vi "Read TDMS waveform --V3.vi"(0 "Input file path":path, 1 "tdms file in":refnum<k34>, 2 "TDMS":T1, 5 "Data window IN":T2={"Start"=39994, "Length"=13169, "Channel numbers"=[0], "Cannel names"=["freq", ""], "Group name"="p"}, 11 "error in":errorcluster) -> (3 "tdms file out":refnum<k34>, 4 "Actual input file path":path, 6 "Data out":waveform(dbl)[](array[waveform]), 8 "All Data out":waveform(dbl)[](array[waveform]), 10 "1st channel length":u64, 15 "error out":errorcluster)   [LabVIEW 2021]
uses:
  fft -- data win.ctl
  Read TDMS waveform -- control.vi.ctl
panel:
  # "OR"
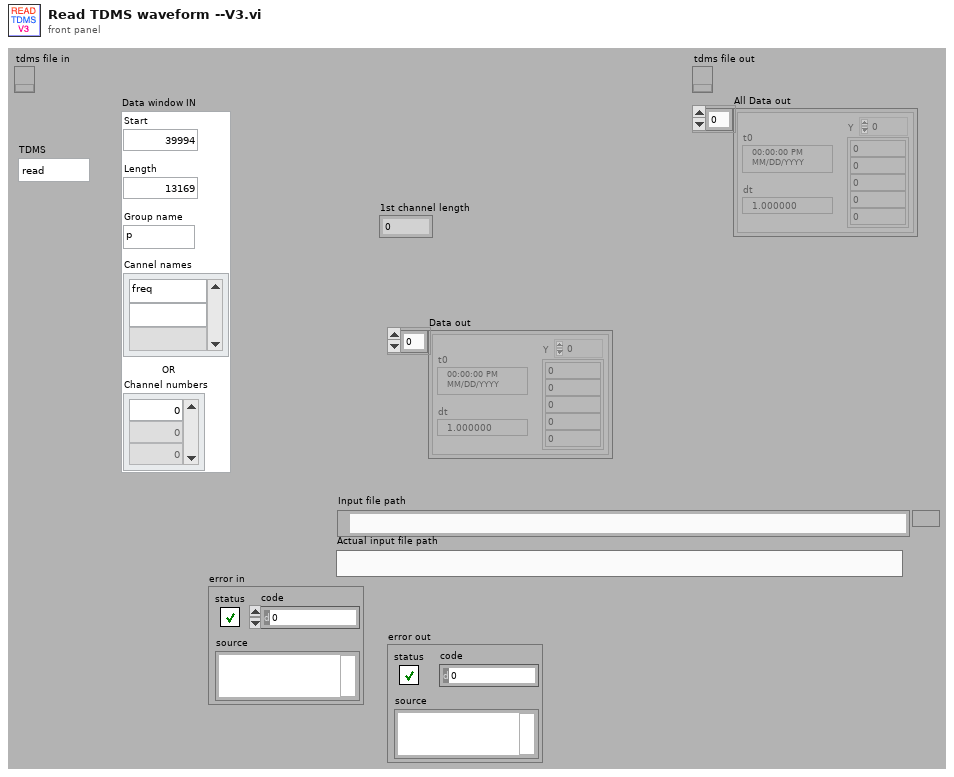
[diagram p1: front panel]
types:
  T1 = typedef "Read TDMS waveform -- control.vi.ctl" = enum16{"read", "open", "close"}
  T2 = typedef "fft -- data win.ctl" = cluster{"Start":i64, "Length":i32, "Channel numbers":i64[], "Cannel names":string[], "Group name":string}
  T3 = enum16{"TDMS file", "Tektronics ISF", "BinF file", "ASCII File", "BinH File", "BinW File", "BINARY File"}
  T4 = enum16{"open", "open or create", "create or replace", "create", "open (read-only)"}
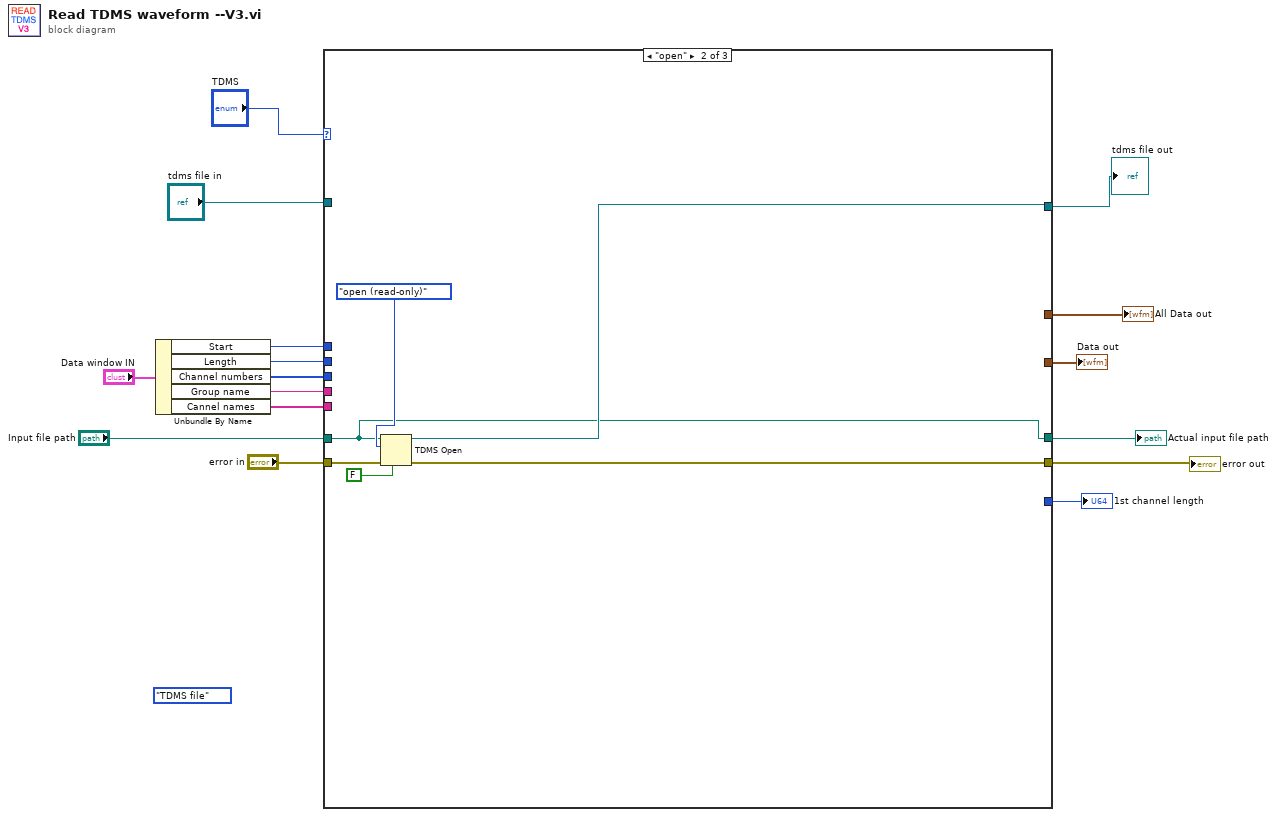
[diagram p0: block diagram]
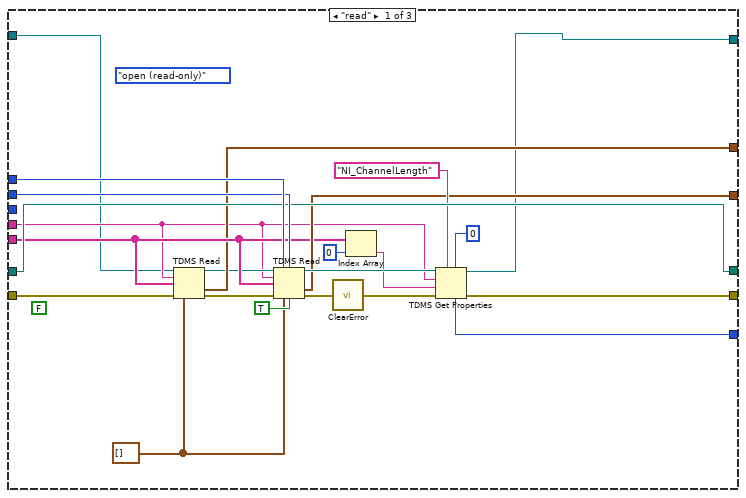
[diagram p2: hidden frame]
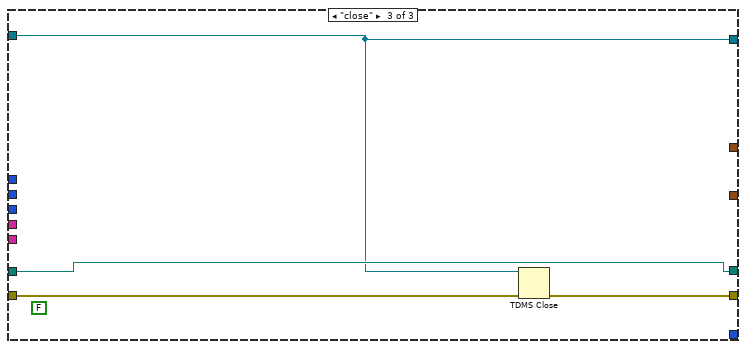
[diagram p3: hidden frame]
diagram:
  (unwired) T3."TDMS file" ("Data File Type")
  n1 = Unbundle By Name("Data window IN") -> ("Start"=w12:i64, "Length"=w11:i32, "Channel numbers"=w13:i64[], "Group name"=w7:string, "Cannel names"=w9:string[])
  n2 = case shown="\"open\"" "TDMS" {
    tunnel: "Input file path" -> [w36 w40 w48]
    tunnel: [w36 w40 w48] -> w15
    tunnel: "error in" -> [w19 w45 w46]
    tunnel: [w18 w41 w49] -> w6
    tunnel: w13 -> [_ _ _]
    tunnel: w12 -> [w39 _ _]
    tunnel: w11 -> [w38 _ _]
    tunnel: [w29 _ _] -> w10
    tunnel: w9 -> [w26 _ _]
    tunnel: [w30 _ _] -> w8
    tunnel: w7 -> [w21 _ _]
    tunnel: [w23 _ _] -> w5
    tunnel: "tdms file in" -> [w20 _ w47]
    tunnel: [w17 w42 w47] -> w1
    frame "read" {
      (unwired) FALSE ("disable buffering (T)")
      (unwired) T4."open (read-only)" ("operation (0:open)")
      w25 = waveform(dbl)[] []
      n3 = TDMS Read(0:w20, 5:w21, 7:w26, 11:w19, 12:w25) -> (4:w22:refnum<k34>, 10:w23:waveform(dbl)[], 15:w24:errorcluster)  [unwired: 3 in, 3 out]
      n4 = TDMS Read(0:w22, 1:w39, 2:w38, 5:w21, 7:w26, 11:w24, 12:w25, 13:TRUE ("return channels in file order? (F)")) -> (4:w35:refnum<k34>, 10:w29:waveform(dbl)[], 15:w28:errorcluster)  [unwired: 3 out]
      n5 = call <vilib>:"ClearError.vi"("error in (no error)"=w28) -> ("error out"=w37:errorcluster)
      n6 = Index Array(array=w26, index=0) -> (element=w33:string)
      n7 = TDMS Get Properties(5:u64 0, 7:"NI_ChannelLength" ("property name"), 8:w37, 9:w33, 10:w21, 11:w35) -> (0:w18:errorcluster, 3:w17:refnum<k34>, 4:w30:u64)  [unwired: 3 out]
    }
    frame "open" {
      n8 = TDMS Open(6:FALSE ("disable buffering (T)"), 8:w45, 10:T4."open (read-only)" ("operation (0:open)"), 11:w40) -> (0:w41:errorcluster, 3:w42:refnum<k34>)  [unwired: 3 in]
    }
    frame "close" {
      (unwired) FALSE ("disable buffering (T)")
      n9 = TDMS Close(8:w46, 11:w47) -> (0:w49:errorcluster)  [unwired: 1 out]
    }
  }
  "Actual input file path" <- w15
  "error out" <- w6
  "Data out" <- w10
  "1st channel length" <- w8
  "tdms file out" <- w1
  "All Data out" <- w5
